vi "test2.vi"() -> ()   [LabVIEW 2019, in "lv-apt-json-file-test.lvlib"]
uses:
  lv-apt-json-file-test.lvlib
  lv-apt-json-file.lvlib
panel:
  out "OrignKey":string
  out "data 3":variant
  out "data 2":variant
  out "data":variant
  out "Cluster":variant
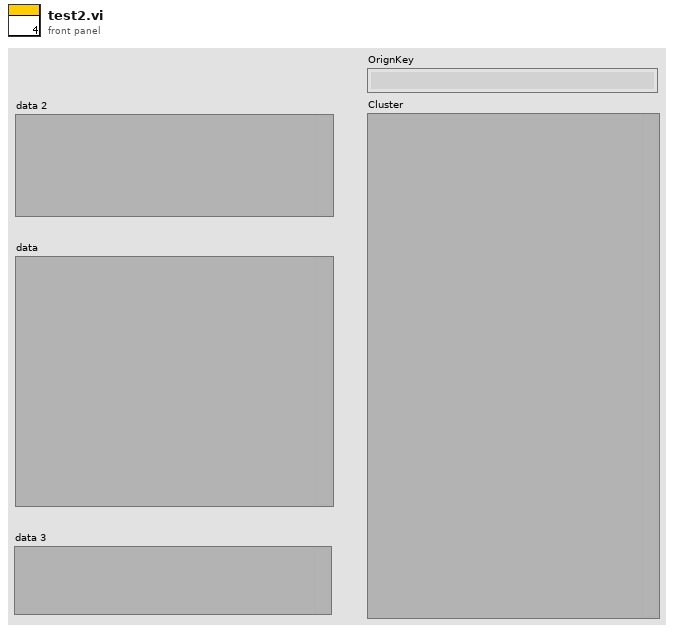
[diagram p1: front panel]
types:
  T1 = cluster{"numeric":i32, "SDDring":string, "Cluster":cluster{"Cumeric":i32, "string":string, "cluster":cluster{"numeric":i32, "string":string, "cluster":cluster{"numeric":i32, "string":string}}}}
  T2 = typedef "lv-apt-json-file.lvlib/Def-AttrMap.ctl" = cluster{"Map":variant}
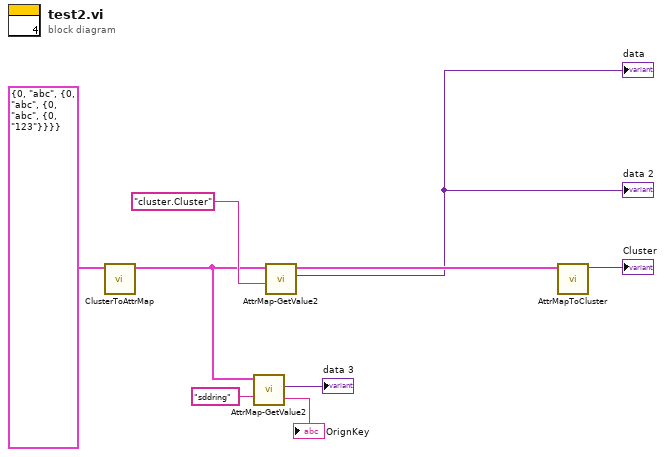
[diagram p0: block diagram]
diagram:
  n1 = call "ClusterToAttrMap.vi"("data"=T1 {"numeric"=0, "SDDring"="abc", "Cluster"={"Cumeric"=0, "string"="abc", "cluster"={"numeric"=0, "string"="abc", "cluster"={"numeric"=0, "string"="123"}}}} ("Cluster")) -> ("AttrMap"=w4:T2)  [unwired: 9 in, 1 out]
  n2 = call "AttrMap-GetValue2.vi"("Key"="sddring", "AttrMap in"=w4) -> ("data"=→"data 3":variant, "OrignKey"=→"OrignKey":string)  [unwired: 6 in, 2 out]
  n3 = call "AttrMap-GetValue2.vi"("Key"="cluster.Cluster", "AttrMap in"=w4) -> ("data"=→"data" →"data 2":variant, "AttrMap out"=w7:T2)  [unwired: 6 in, 2 out]
  n4 = call "AttrMapToCluster.vi"("AttrMap"=w7) -> ("Cluster"=→"Cluster":variant)  [unwired: 9 in, 1 out]
